vi "AudioTest.Load Plot Limit From Config Files.vi"(8 "error in (no error)":errorcluster, 11 "Config Folder":path=path "C:/MTE/Audio Test/Config") -> (0 "error out":errorcluster, 3 "LimitPlots":T1[](array[typedef]))   [LabVIEW 2018]
uses:
  TypeDefs/AudioTest.Result Plot Data.ctl
  <vilib>/KATE/Files/File Utils.lvlib
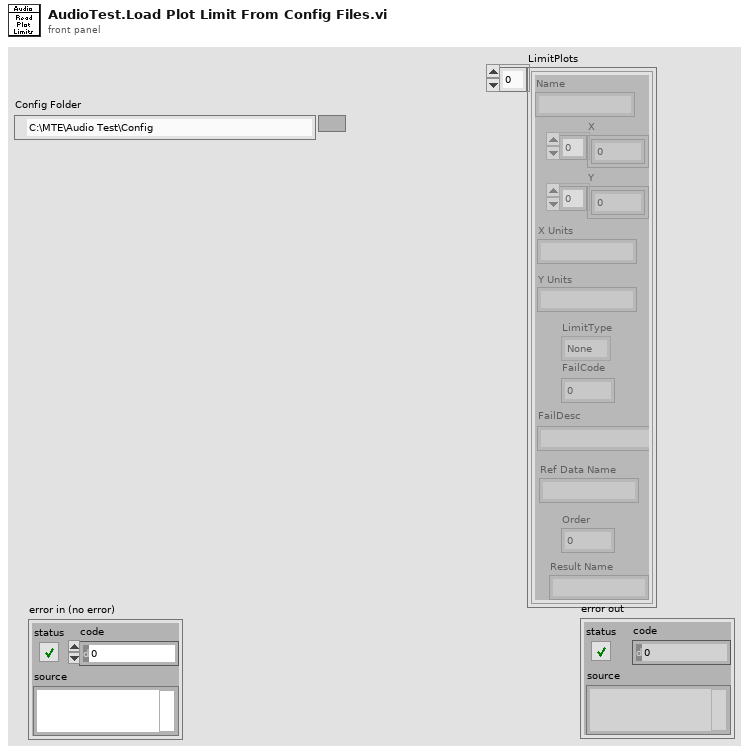
[diagram p1: front panel]
types:
  T1 = typedef "AudioTest.Result Plot Data.ctl" = cluster{"Order":i32, "Name":string, "X":dbl[], "Y":dbl[], "X Units":string, "Y Units":string, "LimitType":enum16{"None", "LL", "UL"}, "FailCode":i32, "FailDesc":string, "Ref Data Name":string, "Result Name":string}
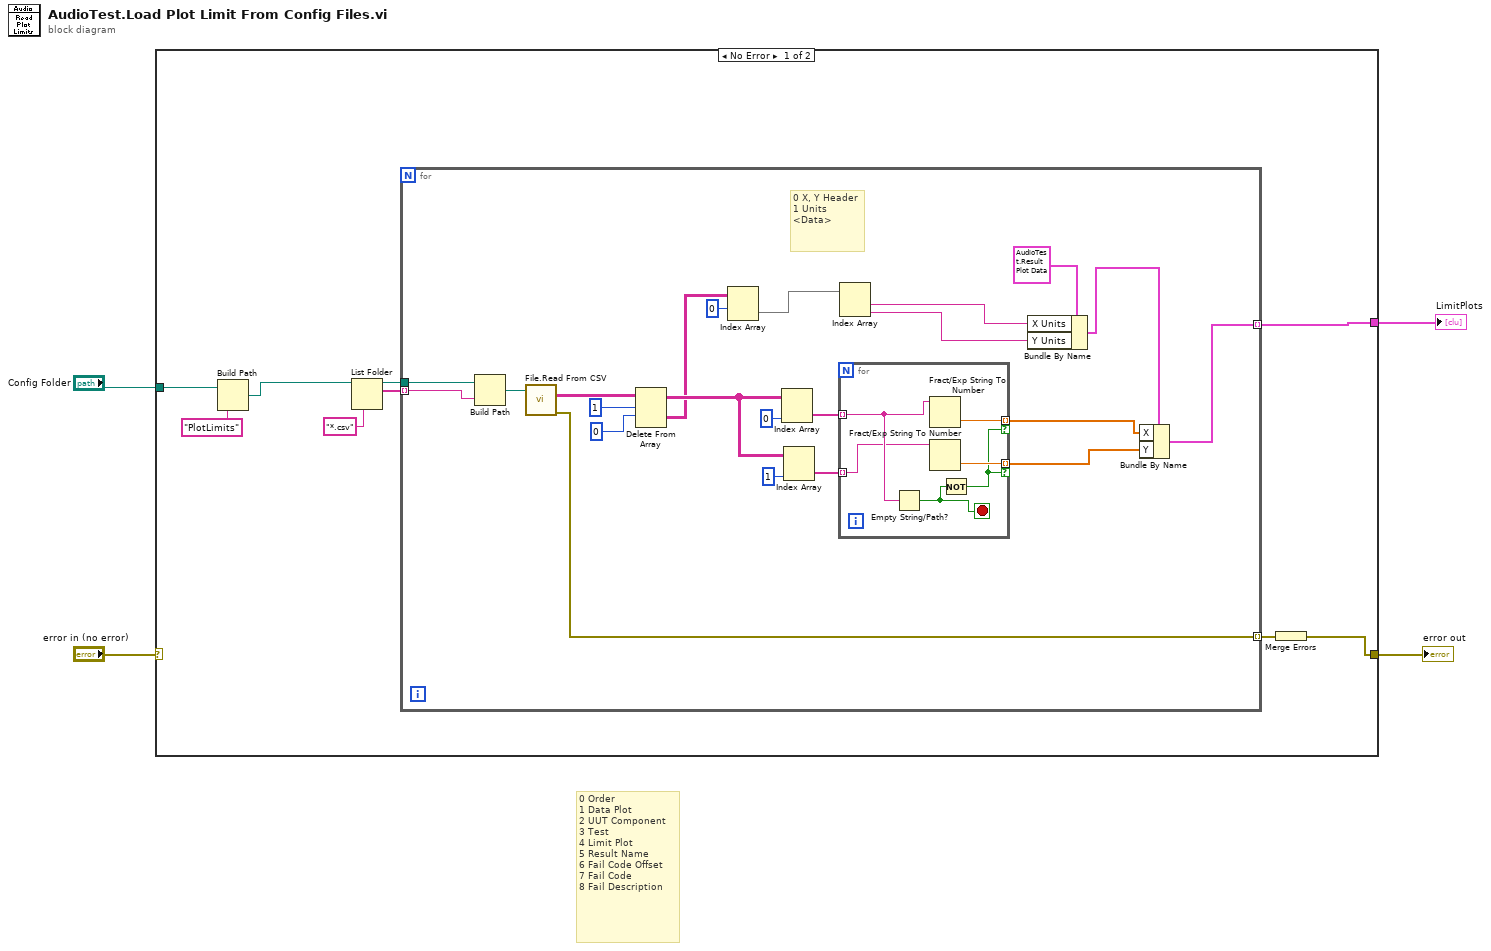
[diagram p0: block diagram]
diagram:
  # "0 Order\n1 Data Plot\n2 UUT Component\n3 Test\n4 Limit Plot\n5 Result Name\n6 Fail Code Offset\n7 Fail Code\n8 Fail Description"
  n1 = case shown="No Error" "error in (no error)" {
    selector: "error in (no error)" -> [_ w42]
    tunnel: "Config Folder" -> [w13 _]
    tunnel: [w7 _] -> w3
    tunnel: [w6 w42] -> w1
    frame No Error {
      n2 = Build Path(base path=w13, name or relative path="PlotLimits") -> (appended path=w11:path)
      n3 = List Folder(path=w11, pattern="*.csv" ("name or relative path")) -> (path out=w9:path, filenames=w8:string[])  [unwired: 2 in, 2 out]
      n4 = for {
        tunnel: w9 -> [w35]
        tunnel: w8 -> [w34] mode=indexing
        tunnel: [w32] -> w5 mode=indexing
        tunnel: [w19] -> w7 mode=indexing
        # "0 X, Y Header\n1 Units\n<Data>"
        n5 = Build Path(base path=w35, name or relative path=w34) -> (appended path=w33:path)
        n6 = call <vilib>:"File.Read From CSV.vi"("File"=w33) -> ("error out"=w32:errorcluster, "Data"=w31:string[][])  [unwired: 8 in, 1 out]
        n7 = Delete From Array(array=w31, length=1, index (row)=0) -> (deleted portion=w16:string[][], array with subset deleted=w25:string[][])  [unwired: 1 in]
        n8 = Index Array(array=w16, index (row)=0) -> (element=w14:string[])  [unwired: 1 in]
        n9 = Index Array(array=w25, index (col)=0 ("disabled index (col)")) -> (element=w24:string[])  [unwired: 1 in]
        n10 = Index Array(array=w25, index (col)=1 ("disabled index (col)")) -> (element=w23:string[])  [unwired: 1 in]
        n11 = for {
          tunnel: w24 -> [w41] mode=indexing
          tunnel: w23 -> [w40] mode=indexing
          tunnel: [w39] -> w20 mode=indexing if=w36
          tunnel: [w38] -> w21 mode=indexing if=w36
          stop <- w37 stop-if-true
          n12 = Empty String/Path?(string/path=w41) -> (empty?=w37:bool)
          n13 = Fract/Exp String To Number(string=w41) -> (number=w38:dbl)  [unwired: 3 in, 1 out]
          n14 = Fract/Exp String To Number(string=w40) -> (number=w39:dbl)  [unwired: 3 in, 1 out]
          n15 = Not(x=w37) -> (.not. x?=w36:bool)
        }
        n16 = Index Array(array=w14) -> (element #1=w17:string, element #2=w18:string)  [unwired: 2 in]
        n17 = Bundle By Name(cluster=T1 {"Order"=0, "Name"="", "X"=[], "Y"=[], "X Units"="", "Y Units"="", "LimitType"=enum."None", "FailCode"=0, "FailDesc"="", "Ref Data Name"="", "Result Name"=""}, "X Units"=w17, "Y Units"=w18) -> (w22:T1)
        n18 = Bundle By Name(cluster=w22, "X"=w21, "Y"=w20) -> (w19:T1)
      }
      n19 = Merge Errors(w5) -> (w6:errorcluster)
    }
    frame Error {
    }
  }
  "LimitPlots" <- w3
  "error out" <- w1
